vi "Main Question.vi"() -> (0 "Question":string[][](array[string])=[["是七人制橄欖球類的運動嗎?", "是男子運動嗎?"], ["是小輪車類的運動嗎?", "是男子運動嗎?"], ["是公路自由車類的運動嗎?", "是男子運動嗎?"], ["是手球類的運動嗎?", "是男子運動嗎?"], ["是水上芭蕾類的運動嗎?", "是團體賽嗎?"], ["是水球類的運動嗎?", "是男子運動嗎?"], ["是田徑類的運動嗎?", "是男子運動嗎?"], ["是划船類的運動嗎?", "是男子運動嗎?"], ["是帆船類的運動嗎?", "是男子運動嗎?"], ["是曲棍球類的運動嗎?", "是男子運動嗎?"], ["是羽球類的運動嗎?", "是男子運動嗎?"], ["是沙灘排球類的運動嗎?", "是男子運動嗎?"], ["是角力類的運動嗎?", "是男子運動嗎?"], ["是足球類的運動嗎?", "是男子運動嗎?"], ["是柔道類的運動嗎?", "是男子運動嗎?"], ["是射箭類的運動嗎?", "是男子運動嗎?"], ["是射擊類的運動嗎?", "是男子運動嗎?"], ["是拳擊類的運動嗎?", "是男子運動嗎?"], ["是桌球類的運動嗎?", "是男子運動嗎?"], ["是馬術類的運動嗎?", "是男子運動嗎?"], ["是高爾夫類的運動嗎?", "是男子運動嗎?"], ["是排球類的運動嗎?", "是男子運動嗎?"], ["是現代五項類的運動嗎?", "是男子運動嗎?"], ["是場地自由車類的運動嗎?", "是男子運動嗎?"], ["是游泳類的運動嗎?", "是男子運動嗎?"], ["是登山自由車類的運動嗎?", "是男子運動嗎?"], ["是跆拳道類的運動嗎?", "是男子運動嗎?"], ["是跳水類的運動嗎?", "是男子運動嗎?"], ["是網球類的運動嗎?", "是男子運動嗎?"], ["是輕艇激流類的運動嗎?", "是男子運動嗎?"], ["是輕艇競速類的運動嗎?", "是男子運動嗎?"], ["是彈翻床類的運動嗎?", "是男子運動嗎?"], ["是擊劍類的運動嗎?", "是男子運動嗎?"], ["是舉重類的運動嗎?", "是男子運動嗎?"], ["是韻律體操類的運動嗎?", "是男子運動嗎?"], ["是競技體操類的運動嗎?", "是男子運動嗎?"], ["是籃球類的運動嗎?", "是男子運動嗎?"], ["是鐵人三項類的運動嗎?", "是男子運動嗎?"]])   [LabVIEW 2015]
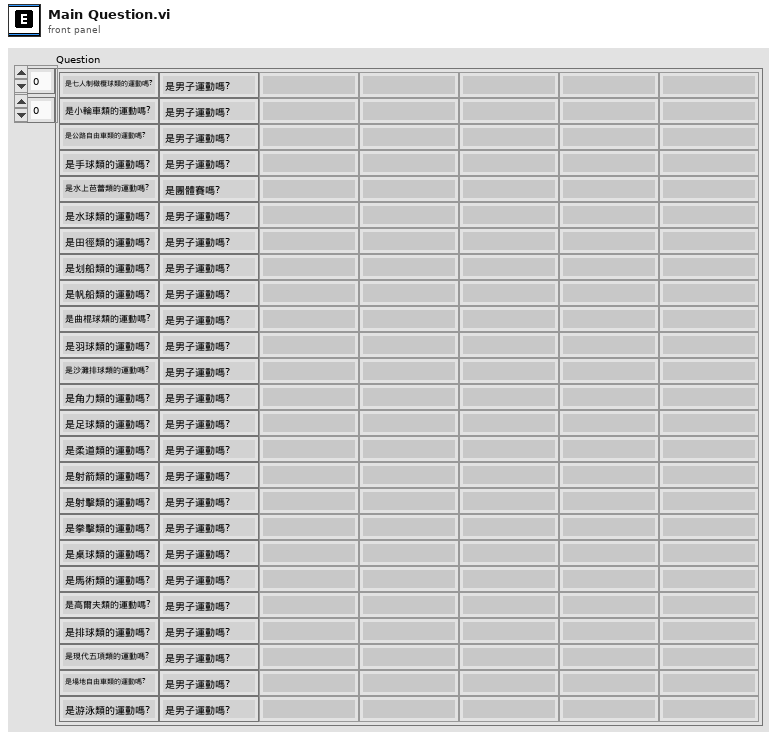
[diagram p1: front panel]
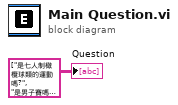
[diagram p0: block diagram]
diagram:
  "Question" <- string[][] [["是七人制橄欖球類的運動嗎?", "是男子賽嗎?", "", "", "", "", "", "", "", "", "", "", "", "", "", "", "", "", "", "", "", "", "", "", "", "", ""], ["是小輪車類的運動嗎?", "是男子賽嗎?", "是計時賽嗎?", "", "", "", "", "", "", "", "", "", "", "", "", "", "", "", "", "", "", "", "", "", "", "", ""], ["是公路自由車類的運動嗎?", "是男子賽嗎?", "", "", "", "", "", "", "", "", "", "", "", "", "", "", "", "", "", "", "", "", "", "", "", "", ""], ["是手球類的運動嗎?", "是男子賽嗎?", "", "", "", "", "", "", "", "", "", "", "", "", "", "", "", "", "", "", "", "", "", "", "", "", ""], ["是水上芭蕾類的運動嗎?", "是團體賽嗎?", "", "", "", "", "", "", "", "", "", "", "", "", "", "", "", "", "", "", "", "", "", "", "", "", ""], ["是水球類的運動嗎?", "是男子賽嗎?", "", "", "", "", "", "", "", "", "", "", "", "", "", "", "", "", "", "", "", "", "", "", "", "", ""], ["是田徑類的運動嗎?", "是男子賽嗎?", "¬O100¤½¤ØÁÉ¶Ü?", "¬O200¤½¤ØÁÉ¶Ü?", "¬O400¤½¤ØÁÉ¶Ü?", "¬O800¤½¤ØÁÉ¶Ü?", "¬O1500¤½¤ØÁÉ¶Ü?", "¬O5000¤½¤ØÁÉ¶Ü?", "¬O10000¤½¤ØÁÉ¶Ü?", "¬O110¤½¤Ø¸óÄæÁÉ¶Ü?", "¬O400¤½¤Ø¸óÄæÁÉ¶Ü?", "¬O3000¤½¤Ø»ÙÃªÁÉ¶Ü?", "¬O4¡Ñ100¤½¤Ø±µ¤OÁÉ¶Ü?", "¬O4¡Ñ400¤½¤Ø±µ¤OÁÉ¶Ü?", "是馬拉松賽嗎?", "¬O20¤½¨½Äv¨«ÁÉ¶Ü?", "¬O50¤½¨½Äv¨«ÁÉ¶Ü?", "是跳高賽嗎?", "¬O¼µ¬ñ¸õÁÉ¶Ü?", "是跳遠賽嗎?", "是三級跳遠賽嗎?", "是鉛球賽嗎?", "是鐵餅賽嗎?", "是鏈球賽嗎?", "是標槍賽嗎?", "是十項全能賽嗎?", "是七項全能賽嗎?"], ["是划船類的運動嗎?", "是男子賽嗎?", "是雙人賽嗎?", "是四人賽嗎?", "是八人賽嗎?", "是單槳賽嗎?", "是雙槳賽嗎?", "是輕量級賽嗎?", "", "", "", "", "", "", "", "", "", "", "", "", "", "", "", "", "", "", ""], ["是帆船類的運動嗎?", "是男子賽嗎?", "¬OX«¬ÁÉ¶Ü?", "是雷射輻射型賽嗎?", "¬O470«¬ÁÉ¶Ü?", "¬O49¤H«¬ÁÉ¶Ü?", "是雷射型賽嗎?", "是芬蘭人型賽嗎?", "是混合Nacra17型賽嗎?", "", "", "", "", "", "", "", "", "", "", "", "", "", "", "", "", "", ""], ["是曲棍球類的運動嗎?", "是男子賽嗎?", "", "", "", "", "", "", "", "", "", "", "", "", "", "", "", "", "", "", "", "", "", "", "", "", ""], ["是羽球類的運動嗎?", "是男子賽嗎?", "是單打賽嗎?", "是混合雙打賽嗎?", "", "", "", "", "", "", "", "", "", "", "", "", "", "", "", "", "", "", "", "", "", "", ""], ["是沙灘排球類的運動嗎?", "是男子賽嗎?", "", "", "", "", "", "", "", "", "", "", "", "", "", "", "", "", "", "", "", "", "", "", "", "", ""], ["是角力類的運動嗎?", "是男子賽嗎?", "是希羅式賽嗎?", "是自由式賽嗎?", "¬O59¤½¤ç¯ÅÁÉ¶Ü?", "¬O66¤½¤ç¯ÅÁÉ¶Ü?", "¬O75¤½¤ç¯ÅÁÉ¶Ü?", "¬O85¤½¤ç¯ÅÁÉ¶Ü?", "¬O98¤½¤ç¯ÅÁÉ¶Ü?", "¬O130¤½¤ç¯ÅÁÉ¶Ü?", "¬O57¤½¤ç¯ÅÁÉ¶Ü?", "¬O65¤½¤ç¯ÅÁÉ¶Ü?", "¬O74¤½¤ç¯ÅÁÉ¶Ü?", "¬O86¤½¤ç¯ÅÁÉ¶Ü?", "¬O97¤½¤ç¯ÅÁÉ¶Ü?", "¬O125¤½¤ç¯ÅÁÉ¶Ü?", "¬O48¤½¤ç¯ÅÁÉ¶Ü?", "¬O53¤½¤ç¯ÅÁÉ¶Ü?", "¬O58¤½¤ç¯ÅÁÉ¶Ü?", "¬O63¤½¤ç¯ÅÁÉ¶Ü?", "¬O69¤½¤ç¯ÅÁÉ¶Ü?", "", "", "", "", "", ""], ["是足球類的運動嗎?", "是男子賽嗎?", "", "", "", "", "", "", "", "", "", "", "", "", "", "", "", "", "", "", "", "", "", "", "", "", ""], ["是柔道類的運動嗎?", "是男子賽嗎?", "¬O60¤½¤ç¯ÅÁÉ¶Ü?", "¬O66¤½¤ç¯ÅÁÉ¶Ü?", "¬O73¤½¤ç¯ÅÁÉ¶Ü?", "¬O81¤½¤ç¯ÅÁÉ¶Ü?", "¬O90¤½¤ç¯ÅÁÉ¶Ü?", "¬O100¤½¤ç¯ÅÁÉ¶Ü?", "¬O100¤½¤ç¥H¤W¯ÅÁÉ¶Ü?", "¬O48¤½¤ç¯ÅÁÉ¶Ü?", "¬O52¤½¤ç¯ÅÁÉ¶Ü?", "¬O57¤½¤ç¯ÅÁÉ¶Ü?", "¬O63¤½¤ç¯ÅÁÉ¶Ü?", "¬O70¤½¤ç¯ÅÁÉ¶Ü?", "¬O78¤½¤ç¯ÅÁÉ¶Ü?", "", "", "", "", "", "", "", "", "", "", "", ""], ["是射箭類的運動嗎?", "是男子賽嗎?", "是個人賽嗎?", "是團體賽嗎?", "", "", "", "", "", "", "", "", "", "", "", "", "", "", "", "", "", "", "", "", "", "", ""], ["是射擊類的運動嗎?", "是男子賽嗎?", "是空氣手槍賽嗎?", "是空氣步槍賽嗎?", "是快射手槍賽嗎?", "是快射手步槍賽嗎?", "是手槍賽嗎?", "¬O¨Bºjª×«ºÁÉ¶Ü?", "¬O¨Bºj¤T«ºÁÉ¶Ü?", "¬O10¤½¤ØÁÉ¶Ü?", "¬O25¤½¤ØÁÉ¶Ü?", "¬O50¤½¤ØÁÉ¶Ü?", "是定向飛靶賽嗎?", "是不定向飛靶賽嗎?", "是雙不定向飛靶賽嗎?", "", "", "", "", "", "", "", "", "", "", "", ""], ["是拳擊類的運動嗎?", "是男子賽嗎?", "是輕蠅量49公斤級賽嗎?", "是蠅量52公斤級賽嗎?", "是雛量56公斤級賽嗎?", "是輕量60公斤級賽嗎?", "是輕沉量64公斤級賽嗎?", "是沉量69公斤級賽嗎?", "是中量75公斤級賽嗎?", "是輕重量81公斤級賽嗎?", "是重量91公斤級賽嗎?", "是超重量91公斤以上級賽嗎?", "是超蠅量51公斤級賽嗎?", "是輕量60公斤級賽嗎?", "是中量75公斤級賽嗎?", "", "", "", "", "", "", "", "", "", "", "", ""], ["是桌球類的運動嗎?", "是男子賽嗎?", "是單打賽嗎?", "", "", "", "", "", "", "", "", "", "", "", "", "", "", "", "", "", "", "", "", "", "", "", ""], ["是馬術類的運動嗎?", "是團體賽嗎?", "是盛裝舞步賽嗎?", "是三項賽嗎?", "", "", "", "", "", "", "", "", "", "", "", "", "", "", "", "", "", "", "", "", "", "", ""], ["是高爾夫類的運動嗎?", "是男子賽嗎?", "", "", "", "", "", "", "", "", "", "", "", "", "", "", "", "", "", "", "", "", "", "", "", "", ""], ["是排球類的運動嗎?", "是男子賽嗎?", "", "", "", "", "", "", "", "", "", "", "", "", "", "", "", "", "", "", "", "", "", "", "", "", ""], ["是現代五項類的運動嗎?", "是男子賽嗎?", "", "", "", "", "", "", "", "", "", "", "", "", "", "", "", "", "", "", "", "", "", "", "", "", ""], ["是場地自由車類的運動嗎?", "是男子賽嗎?", "是團體賽嗎?", "是爭先賽嗎?", "是追逐賽嗎?", "", "", "", "", "", "", "", "", "", "", "", "", "", "", "", "", "", "", "", "", "", ""], ["是游泳類的運動嗎?", "是男子賽嗎?", "¬O±¶ªaÁÉ¶Ü?", "是仰式賽嗎?", "是蛙式賽嗎?", "是蝶式賽嗎?", "是混合式賽嗎?", "是接力賽嗎?", "是公開水域賽嗎?", "", "", "", "", "", "", "", "", "", "", "", "", "", "", "", "", "", ""], ["是登山自由車類的運動嗎?", "是男子賽嗎?", "", "", "", "", "", "", "", "", "", "", "", "", "", "", "", "", "", "", "", "", "", "", "", "", ""], ["是跆拳道類的運動嗎?", "是男子賽嗎?", "¬O68¤½¤ç¯ÅÁÉ¶Ü?", "¬O80¤½¤ç¯ÅÁÉ¶Ü?", "¬O80¤½¤ç¥H¤W¯ÅÁÉ¶Ü?", "¬O49¤½¤ç¯ÅÁÉ¶Ü?", "¬O57¤½¤ç¯ÅÁÉ¶Ü?", "¬O67¤½¤ç¯ÅÁÉ¶Ü?", "¬O67¤½¤ç¥H¤W¯ÅÁÉ¶Ü?", "", "", "", "", "", "", "", "", "", "", "", "", "", "", "", "", "", ""], ["是跳水類的運動嗎?", "是男子賽嗎?", "是跳板賽嗎?", "是跳台賽嗎?", "¬O3¤½¤ØÁÉ¶Ü?", "¬O10¤½¤ØÁÉ¶Ü?", "是雙人賽嗎?", "", "", "", "", "", "", "", "", "", "", "", "", "", "", "", "", "", "", "", ""], ["是網球類的運動嗎?", "是男子賽嗎?", "是單打賽嗎?", "是混合雙打賽嗎?", "", "", "", "", "", "", "", "", "", "", "", "", "", "", "", "", "", "", "", "", "", "", ""], ["是輕艇激流類的運動嗎?", "是男子賽嗎?", "是加拿大式艇嗎?", "是愛斯基摩艇嗎?", "", "", "", "", "", "", "", "", "", "", "", "", "", "", "", "", "", "", "", "", "", "", ""], ["是輕艇競速類的運動嗎?", "是男子賽嗎?", "是雙人賽嗎?", "是加拿大式艇嗎?", "是愛斯基摩艇嗎?", "¬O200¤½¤ØÁÉ¶Ü?", "¬O1000¤½¤ØÁÉ¶Ü?", "¬O500¤½¤ØÁÉ¶Ü?", "", "", "", "", "", "", "", "", "", "", "", "", "", "", "", "", "", "", ""], ["是彈翻床類的運動嗎?", "是男子賽嗎?", "", "", "", "", "", "", "", "", "", "", "", "", "", "", "", "", "", "", "", "", "", "", "", "", ""], ["是擊劍類的運動嗎?", "是男子賽嗎?", "是團體賽嗎?", "¬O¶w¼CÁÉ¶Ü?", "¬O¾U¼CÁÉ¶Ü?", "是軍刀賽嗎?", "", "", "", "", "", "", "", "", "", "", "", "", "", "", "", "", "", "", "", "", ""], ["是舉重類的運動嗎?", "是男子賽嗎?", "¬O56¤½¤ç¯ÅÁÉ¶Ü?", "¬O62¤½¤ç¯ÅÁÉ¶Ü?", "¬O69¤½¤ç¯ÅÁÉ¶Ü?", "¬O77¤½¤ç¯ÅÁÉ¶Ü?", "¬O85¤½¤ç¯ÅÁÉ¶Ü?", "¬O94¤½¤ç¯ÅÁÉ¶Ü?", "¬O105¤½¤ç¯ÅÁÉ¶Ü?", "¬O105¤½¤ç¥H¤W¯ÅÁÉ¶Ü?", "¬O105¤½¤ç¥H¤W¯ÅÁÉ¶Ü?", "¬O48¤½¤ç¯ÅÁÉ¶Ü?", "¬O53¤½¤ç¯ÅÁÉ¶Ü?", "¬O58¤½¤ç¯ÅÁÉ¶Ü?", "¬O63¤½¤ç¯ÅÁÉ¶Ü?", "¬O69¤½¤ç¯ÅÁÉ¶Ü?", "¬O75¤½¤ç¯ÅÁÉ¶Ü?", "¬O75¤½¤ç¥H¤W¯ÅÁÉ¶Ü?", "", "", "", "", "", "", "", "", ""], ["是韻律體操類的運動嗎?", "是團體賽嗎?", "是雙人賽嗎?", "是四人賽嗎?", "", "", "", "", "", "", "", "", "", "", "", "", "", "", "", "", "", "", "", "", "", "", ""], ["是競技體操類的運動嗎?", "是男子賽嗎?", "是團體賽嗎?", "是跳馬賽嗎?", "是自由體操賽嗎?", "是鞍馬賽嗎?", "是吊環賽嗎?", "是雙槓賽嗎?", "是單槓賽嗎?", "是全能競技體操賽嗎?", "是平衡木賽嗎?", "是高低槓賽嗎?", "", "", "", "", "", "", "", "", "", "", "", "", "", "", ""], ["是籃球類的運動嗎?", "是男子賽嗎?", "", "", "", "", "", "", "", "", "", "", "", "", "", "", "", "", "", "", "", "", "", "", "", "", ""], ["是鐵人三項類的運動嗎?", "是男子賽嗎?", "", "", "", "", "", "", "", "", "", "", "", "", "", "", "", "", "", "", "", "", "", "", "", "", ""]] ("Table of Data")
